vi "DC.vi"(2 "C":bool, 3 "D":bool) -> (0 "nQ":bool, 1 "Q":bool)   [LabVIEW 2017]
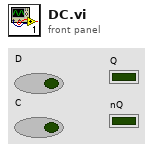
[diagram p1: front panel]
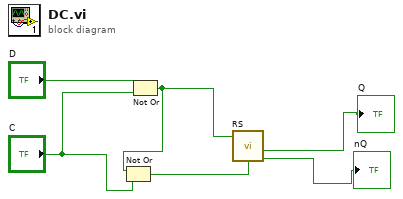
[diagram p0: block diagram]
diagram:
  n1 = Not Or(1:"C", 2:"D") -> (0:w4:bool)
  n2 = Not Or(1:"C", 2:w4) -> (0:w3:bool)
  n3 = call "RS.vi"("S"=w3, "R"=w4) -> ("nQ"=→"nQ":bool, "Q"=→"Q":bool)
